vi "Read DeviceMessages.vi"(8 "error in (no error)":errorcluster, 11 "CS++ControllerActor in":refnum<class "CS++ControllerActor.lvclass">) -> (0 "error out":errorcluster, 2 "DeviceMessages":T1(array[cluster]), 3 "CS++ControllerActor out":refnum<class "CS++ControllerActor.lvclass">)   [LabVIEW 2014, in "CS++ControllerActor.lvlib" / "CS++ControllerActor.lvclass"]
uses:
  CS++ControllerActor.lvclass
  CS++PVMonitor Messages/CS++PVUpdate Msg/CS++PVUpdate Msg.lvclass
  Classes/CS++ProcessVariables/PVConnection/PVConnection.lvclass
  CS++ControllerActor.lvclass/CS++ControllerActor.ctl
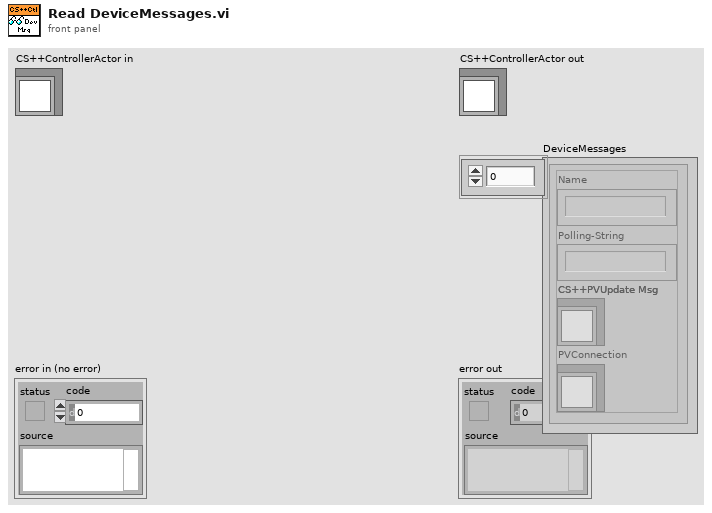
[diagram p1: front panel]
types:
  T1 = cluster{"Name":string, "Polling-String":string, "CS++PVUpdate Msg":refnum<class "CS++PVUpdate Msg.lvclass">, "PVConnection":refnum<class "PVConnection.lvclass">}[]
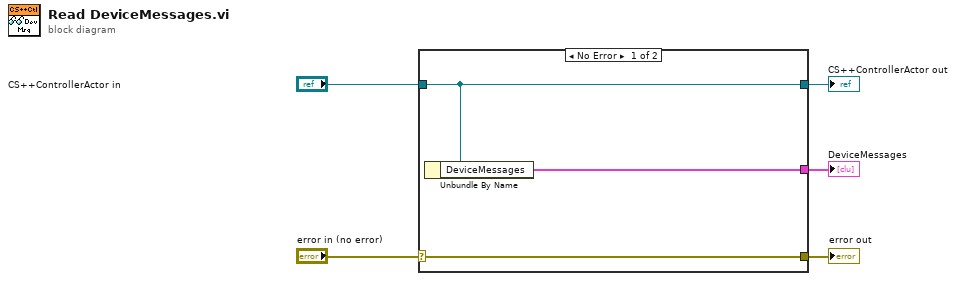
[diagram p0: block diagram]
diagram:
  n1 = case shown="No Error" "error in (no error)" {
    selector: "error in (no error)" -> [w8 w9]
    tunnel: [w8 w9] -> w4
    tunnel: [w7 w10] -> w2
    tunnel: "CS++ControllerActor in" -> [w7 w10]
    tunnel: [w6 _] -> w1
    frame No Error {
      n2 = Unbundle By Name(w7) -> ("DeviceMessages"=w6:T1)
    }
    frame Error {
    }
  }
  "error out" <- w4
  "CS++ControllerActor out" <- w2
  "DeviceMessages" <- w1
